vi "Generate UUID.vi"(8 "error in (no error)":errorcluster) -> (0 "error out":errorcluster, 2 "Binairy UUID":u8[](array[numeric]) format="%02x", 3 "String UUID":string)   [LabVIEW 2018, in "Actor Nest.lvlib" / "Actor Nest.lvclass"]
doc: "This VI calculates a version 4 UUID from pseudo random numbers according to RFC 4122.\n\nFor details see:\nhttp://tools.ietf.org/html/rfc4122"
uses:
  Actor Nest.lvclass
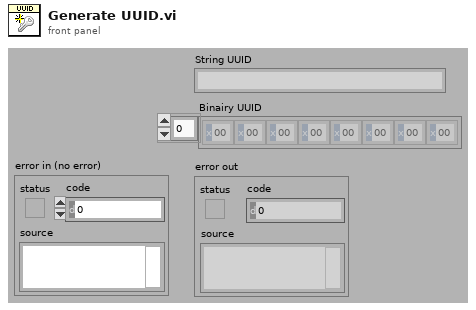
[diagram p1: front panel]
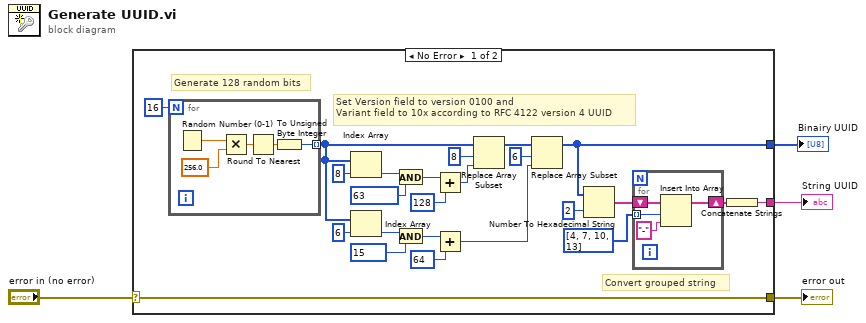
[diagram p0: block diagram]
diagram:
  n1 = case shown="No Error" "error in (no error)" {
    selector: "error in (no error)" -> [w5 w38]
    tunnel: [w7 _] -> w4
    tunnel: [w5 w38] -> w3
    tunnel: [w6 _] -> w1
    frame No Error {
      # "Convert grouped string"
      # "Set Version field to version 0100 and \nVariant field to 10x according to RFC 4122 version 4 UUID"
      # "Generate 128 random bits"
      n2 = for {
        N: 16 -> [_]
        tunnel: [w33] -> w23 mode=indexing
        n3 = Random Number (0-1)() -> (number: 0 to 1=w37:dbl)
        n4 = Multiply(x=w37, y=256.0) -> (x*y=w35:dbl)
        n5 = Round To Nearest(number=w35) -> (nearest integer value=w34:dbl)
        n6 = To Unsigned Byte Integer(number=w34) -> (unsigned 8bit integer=w33:u8)
      }
      n7 = Index Array(array=w23, index=8) -> (element=w26:u8)
      n8 = Index Array(array=w23, index=6) -> (element=w19:u8)
      n9 = And(x=w26, y=u8 63) -> (x .and. y?=w10:u8)
      n10 = And(x=w19, y=u8 15) -> (x .and. y?=w17:u8)
      n11 = Add(x=w10, y=u8 128) -> (x+y=w9:u8)
      n12 = Add(x=w17, y=u8 64) -> (x+y=w15:u8)
      n13 = Replace Array Subset(array=w23, new element=w9, index=8) -> (w21:u8[])
      n14 = Replace Array Subset(array=w21, new element=w15, index=6) -> (w6:u8[])
      n15 = Number To Hexadecimal String(1:i16 2 ("width (-)"), 2:w6) -> (0:w13:string[])
      n16 = for {
        shift-right: [w31] -> w12
        shift-left: w13 -> [w32]
        tunnel: i32[] [4, 7, 10, 13] ("Array") -> [w29] mode=indexing
        n17 = Insert Into Array(array=w32, index=w29, new element="-" ("new element/subarray")) -> (w31:string[])
      }
      n18 = Concatenate Strings(w12) -> (w7:string)
    }
    frame Error {
    }
  }
  "String UUID" <- w4
  "error out" <- w3
  "Binairy UUID" <- w1
